vi "publishIntensityEvnt.vi"(8 "error in (no error)":errorcluster, 10 "Intensity":dbl format="%#_13g", 11 "Electrometer in":refnum<class "Electrometer.lvclass">) -> (0 "error out":errorcluster, 2 "Intensity out":dbl, 3 "Electrometer out":refnum<class "Electrometer.lvclass">)   [LabVIEW 2016, in "Electrometer.lvclass"]
uses:
  Electrometer.lvclass
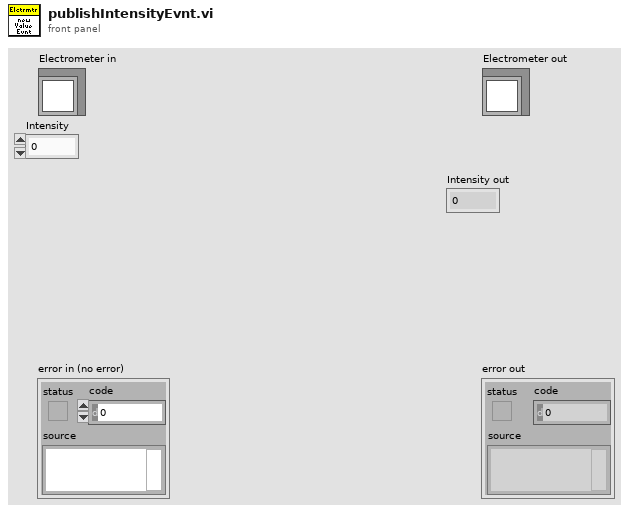
[diagram p1: front panel]
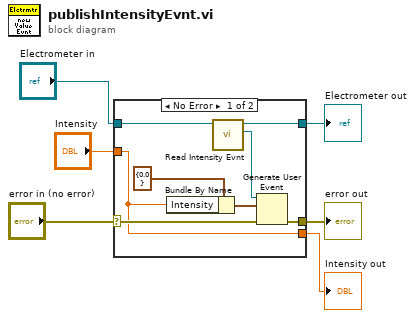
[diagram p0: block diagram]
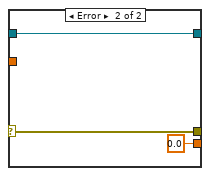
[diagram p2: hidden frame]
diagram:
  n1 = case shown="No Error" "error in (no error)" {
    selector: "error in (no error)" -> [w10 w17]
    tunnel: [w9 w17] -> w5
    tunnel: [w8 w16] -> w3
    tunnel: "Electrometer in" -> [w12 w16]
    tunnel: "Intensity" -> [w7 _]
    tunnel: [w7 0.0 ("Intensity")] -> w1
    frame No Error {
      n2 = Bundle By Name(cluster=cluster{"Intensity":dbl} {"Intensity"=0.0} ("event data"), "Intensity"=w7) -> (w13:cluster{"Intensity":dbl})
      n3 = call-dynamic "Read Intensity Evnt.vi"("Electrometer in"=w12) -> ("Intensity"=w11:refnum<user-event>, "Electrometer out"=w8:refnum<class "Electrometer.lvclass">)  [unwired: 8 in, 1 out]
      n4 = Generate User Event(user event=w11, event data cluster=w13, error in=w10) -> (error out=w9:errorcluster)  [unwired: 1 in, 1 out]
    }
    frame Error {
    }
  }
  "error out" <- w5
  "Electrometer out" <- w3
  "Intensity out" <- w1
